vi "left_centrolize_v2.vi"(0 "samples":i32, 1 "step(mm)":i32, 2 "inner_b_ir":dbl, 3 "inner_f_ir":dbl) -> ()   [LabVIEW 2017]
uses:
  <vilib>/myRIO/Instrument Drivers/Onboard IO/AI/typedefs/AI Reference.ctl
  <vilib>/myRIO/Common/Instrument Driver Framework/Utilities/typedefs/myRIO Generic Hardware Reference.ctl
  <vilib>/myRIO/Common/Instrument Driver Framework/Utilities/typedefs/Hardware Version Enum.ctl
  <vilib>/myRIO/Common/Instrument Driver Framework/Utilities/typedefs/myRIO v1.0 Reference.ctl
  <vilib>/myRIO/Common/Instrument Driver Framework/Utilities/typedefs/Generic FPGA Reference.ctl
  <vilib>/myRIO/Common/Instrument Driver Framework/myRIO v1.0/AI/typedefs/AI Channels List.ctl
  <vilib>/myRIO/Common/Instrument Driver Framework/myRIO v1.0/AI/typedefs/AI Channels Enum.ctl
  <vilib>/myRIO/Common/Instrument Driver Framework/Utilities/typedefs/Analog Scaling Constants List.ctl
  <vilib>/myRIO/Common/Instrument Driver Framework/Utilities/typedefs/Analog Scaling Constants.ctl
  <vilib>/userdefined/High Color/nirio_resource_hc.ctl
  <vilib>/myRIO/Common/Instrument Driver Framework/Utilities/vis/Is FPGA Ref Available.vi
  <vilib>/myRIO/Common/Instrument Driver Framework/myRIO v1.0/AI/vis/myRIO v1.1 Open AI.vi
  <vilib>/myRIO/Instrument Drivers/Onboard IO/AI/vis/Read.vi
  <vilib>/Analysis/baseanly.llb/Mean (DBL).vi
  <vilib>/myRIO/Common/Instrument Driver Framework/Utilities/vis/Validate Channels.vi
  <vilib>/myRIO/Common/Instrument Driver Framework/myRIO v1.0/AI/vis/myRIO v1.0 Reserve AI.vi
  <vilib>/myRIO/Common/Instrument Driver Framework/myRIO v1.0/AI/vis/myRIO v1.0 Build MUX Configuration AI.vi
  <vilib>/myRIO/Common/Instrument Driver Framework/myRIO v1.0/Resource Manager/vis/myRIO v1.0 Reserve Channel List.vi
  <vilib>/myRIO/Common/Instrument Driver Framework/myRIO v1.0/Resource Manager/vis/myRIO v1.0 Reserve Channel.vi
  <vilib>/myRIO/Common/Instrument Driver Framework/myRIO v1.0/Resource Manager/vis/myRIO v1.0 Unreserve Channel.vi
  <vilib>/myRIO/Common/Instrument Driver Framework/myRIO v1.0/Resource Manager/vis/myRIO v1.0 Build Mutex Name.vi
  <vilib>/Utility/VariantDataType/GetNumericInfo.vi
  <vilib>/Utility/error.llb/Error Cluster From Error Code.vi
  <vilib>/myRIO/Common/Instrument Driver Framework/myRIO v1.0/myRIO v1.1 Open.vi
  <vilib>/myRIO/Common/Instrument Driver Framework/myRIO v1.0/AI/vis/myRIO v1.0 Get Scaling Constants AI.vi
  <vilib>/myRIO/Common/Instrument Driver Framework/Utilities/vis/IO Manager.vi
  <vilib>/myRIO/Common/Instrument Driver Framework/Utilities/vis/Configuration Manager.vi
  <vilib>/myRIO/Common/Instrument Driver Framework/myRIO v1.0/myRIO v1.0 Close.vi
  <vilib>/myRIO/Common/Instrument Driver Framework/myRIO v1.0/AI/vis/myRIO v1.0 Read AI.vi
  GlobalVar.vi
  <vilib>/myRIO/Express VI/Onboard IO/AI/AI Express VI.xnode
  <vilib>/myRIO/Instrument Drivers/Onboard IO/AI/vis/myRIO AI Open.xnode
  <vilib>/myRIO/Instrument Drivers/Onboard IO/AI/AI.lvlib
  <vilib>/Analysis/NI_AALBase.lvlib
panel:
  out "pre_r":i32
  out "pre_l":i32
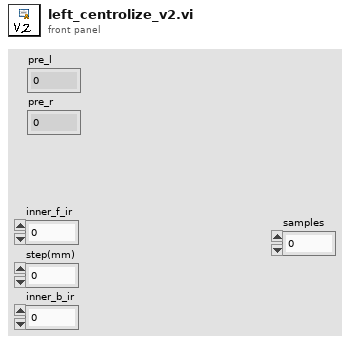
[diagram p1: front panel]
types:
  T1 = typedef "AI.lvlib/AI Reference.ctl" = cluster{"myRIO Reference":T2, "AI Channels List":T6, "AI Scaling Constants List":T8}
  T2 = typedef "myRIO Generic Hardware Reference.ctl" = cluster{"myRIO Model":T3, "myRIO Hardware Reference":T4}
  T3 = typedef "Hardware Version Enum.ctl" = enum16{"Unknown", "myRIO-1900", "myRIO-1950", "roboRIO", "NI ELVIS RIO CM"}
  T4 = typedef "myRIO v1.0 Reference.ctl" = cluster{"Generic FPGA Reference":T5, "Allow multiple opens":bool}
  T5 = typedef "Generic FPGA Reference.ctl" = refnum<k20>
  T6 = typedef "AI Channels List.ctl" = T7[]
  T7 = typedef "AI Channels Enum.ctl" = enum16{"Not Connected", "AudioIn/Left", "AudioIn/Right", "C/AI0", "C/AI1", "A/AI0", "A/AI1", "A/AI2", "A/AI3", "B/AI0", "B/AI1", "B/AI2", "B/AI3", "AI/AI0", "AI/AI1", "AI/AI2", "AI/AI3"}
  T8 = typedef "Analog Scaling Constants List.ctl" = T9[]
  T9 = typedef "Analog Scaling Constants.ctl" = cluster{"LSB Weight (Volts)":dbl, "Offset (Volts)":dbl, "Signed?":bool}
  T10 = typedef "nirio_resource_hc.ctl" = tag
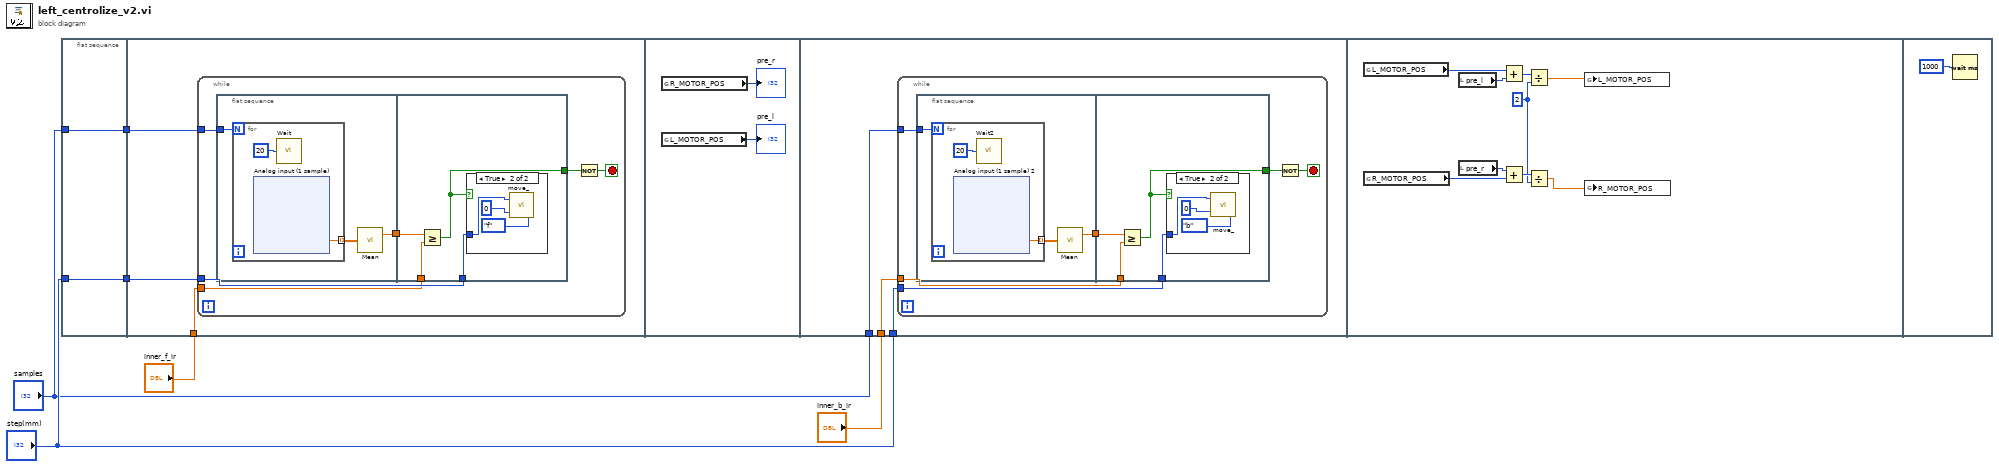
[diagram p0: block diagram]
diagram:
  n1 = flat-sequence {
    tunnel: "step(mm)" -> [w7]
    tunnel: "samples" -> [w8]
    tunnel: [w8] -> w3
    tunnel: [w7] -> w2
    tunnel: w3 -> [w11]
    tunnel: w2 -> [w10]
    tunnel: "inner_f_ir" -> [w9]
    tunnel: "step(mm)" -> [w71]
    tunnel: "inner_b_ir" -> [w70]
    tunnel: "samples" -> [w69]
    frame #0 {
    }
    frame #1 {
      n2 = while {
        tunnel: w11 -> [w17]
        tunnel: w10 -> [w15]
        tunnel: w9 -> [w12]
        stop <- w14 stop-if-true
        n3 = flat-sequence {
          tunnel: w17 -> [w19]
          tunnel: [w18] -> w16
          tunnel: w16 -> [w63]
          tunnel: w15 -> [w62]
          tunnel: [w61] -> w13
          tunnel: w12 -> [w60]
          frame #0 {
            n4 = for {
              N: w19 -> [_]
              tunnel: [w22] -> w20 mode=indexing
              n5 = xnode "Analog input (1 sample)"() -> ("lf (B/AI2 (Pin 7))"=w22:dbl)  [unwired: 1 in, 1 out]
              n6 = call "Wait"("Count(uSec)"=u32 20) -> ()  [unwired: 1 out]
            }
            n7 = call-poly <vilib>:"Mean.vi"("X"=w20) -> ("mean"=w18:dbl)  [unwired: 1 out]
          }
          frame #1 {
            n8 = Greater Or Equal?(x=w63, y=w60) -> (x >= y?=w61:bool)
            n9 = case shown="True" w61 {
              tunnel: w62 -> [_ w66]
              frame False {
              }
              frame True {
                n10 = call "move_.vi"("Enum"=enum16{"hold", "f", "b"}."f", "delay"=u32 0, "D"=w66) -> ()  [unwired: 1 in]
              }
            }
          }
        }
        n11 = Not(x=w13) -> (.not. x?=w14:bool)
      }
    }
    frame #2 {
      n12 = global read "GlobalVar.vi" "R_MOTOR_POS"() -> (→"pre_r":i32)
      n13 = global read "GlobalVar.vi" "L_MOTOR_POS"() -> (→"pre_l":i32)
    }
    frame #3 {
      n14 = while {
        tunnel: w71 -> [w76]
        tunnel: w70 -> [w73]
        tunnel: w69 -> [w72]
        stop <- w75 stop-if-true
        n15 = flat-sequence {
          tunnel: [w80] -> w77
          tunnel: w72 -> [w78]
          tunnel: w77 -> [w123]
          tunnel: w76 -> [w122]
          tunnel: [w121] -> w74
          tunnel: w73 -> [w120]
          frame #0 {
            n16 = for {
              N: w78 -> [_]
              tunnel: [w82] -> w79 mode=indexing
              n17 = xnode "Analog input (1 sample) 2"() -> ("lb (B/AI3 (Pin 9))"=w82:dbl)  [unwired: 1 in, 1 out]
              n18 = call "Wait2"("Count(uSec)"=u32 20) -> ()  [unwired: 1 out]
            }
            n19 = call-poly <vilib>:"Mean.vi"("X"=w79) -> ("mean"=w80:dbl)  [unwired: 1 out]
          }
          frame #1 {
            n20 = Greater Or Equal?(x=w123, y=w120) -> (x >= y?=w121:bool)
            n21 = case shown="True" w121 {
              tunnel: w122 -> [_ w126]
              frame False {
              }
              frame True {
                n22 = call "move_.vi"("Enum"=enum16{"hold", "f", "b"}."b", "delay"=u32 0, "D"=w126) -> ()  [unwired: 1 in]
              }
            }
          }
        }
        n23 = Not(x=w74) -> (.not. x?=w75:bool)
      }
    }
    frame #4 {
      w129 = 2 ("y")
      n24 = global read "GlobalVar.vi" "L_MOTOR_POS"() -> (w135:i32)
      n25 = global read "GlobalVar.vi" "R_MOTOR_POS"() -> (w134:i32)
      n26 = local read "pre_l"() -> (w133:i32)
      n27 = local read "pre_r"() -> (w132:i32)
      n28 = Add(x=w135, y=w133) -> (x+y=w131:i32)
      n29 = Add(x=w132, y=w134) -> (x+y=w130:i32)
      n30 = Divide(x=w131, y=w129) -> (x/y=w127:dbl)
      n31 = Divide(x=w130, y=w129) -> (x/y=w128:dbl)
      n32 = global write "GlobalVar.vi" "L_MOTOR_POS"(w127) -> ()
      n33 = global write "GlobalVar.vi" "R_MOTOR_POS"(w128) -> ()
    }
    frame #5 {
      n34 = Wait (ms)(milliseconds to wait=u32 1000) -> ()  [unwired: 1 out]
    }
  }
